vi "Big_LED_control.vi"() -> ()   [LabVIEW 2018]
uses:
  C:/Users/user/Desktop/LabVIEW/LED_CONTROL_big/LED_CONTROL_big_LED_ophir/AT lib/AmateurStepperMotor.dll
  AT lib/AmateurStepperMotor.dll
  <instrlib>/niDMM/nidmm.llb/niDMM Function.ctl
  <instrlib>/niDMM/nidmm.llb/niDMM Resolution in Digits.ctl
  <instrlib>/niDCPower/nidcpower.llb/niDCPower Measurement Type.ctl
  <vilib>/Instr/_visa.llb/VISA Configure Serial Port (Instr).vi
  <instrlib>/niDMM/nidmm.llb/niDMM Configure Measurement Digits.vi
panel:
  in  "Tab Control":T1(tab)
  in  "POWER":bool
  in  "Стоп":bool
  in  "Resource Name":refnum<k15>="PXI1Slot2" caption="Источник питания"
  in  "Амперметр":refnum<k15>="PXI1Slot5" caption="NI DMM 1"
  in  "V_MB, V":dbl=5.0 caption="voltage level" format="%_6p"
  in  "curlim_V_MB, A":dbl=0.3 caption="current limit" format="%_6p"
  in  "curlim_V_RESERVE, A":dbl=0.1 caption="current limit" min=0.01 format="%_6p"
  out "currentmes_V_MB, A":dbl caption="measurement" format="%_6g"
  out "currentmes_V_RESERVE, A":dbl caption="measurement" format="%_6g"
  in  "V_RESERVE, V":dbl caption="voltage level" format="%_6p"
  out "chart_2":dbl(graph)=8.556104343922883e-07
  out "chart_0":dbl(graph)=5.42616690347781e-05 caption="Waveform Chart 5"
  in  "curlim_V_LED, A":dbl=0.01 caption="current limit" min=0.01 format="%_6p"
  in  "V_LED, V":dbl=2.000000000000001 caption="voltage level" format="%_6p"
  out "chart_1":dbl(graph)=2.456762028615791e-06 caption="Waveform Chart 5"
  out "currentmes_V_LED, A":dbl caption="measurement" format="%_6g"
  in  "NI DMM 1 Current Range 3":string(combo)="1" caption="Range"
  in  "NI DMM 1 units 3":string(combo)="1000" caption="Units"
  out "Current Char":dbl(graph)=0.013612861948786303
  out "Current":dbl format="%_6g"
  in  "Arduino":refnum<visa-resource-name>="COM14"
  in  "Сегменты":bool[](array[boolean])=[FALSE, FALSE, FALSE, FALSE, FALSE, FALSE, FALSE, FALSE, FALSE, FALSE]
  in  "Вольтметр":refnum<k15>="PXI1Slot5" caption="NI DMM 1"
  in  "NI DMM 1 Voltage Range 4":string(combo)="-1" caption="Range"
  out "Voltage Char":dbl(graph)=0.013612861948786303
  in  "NI DMM 1 units 4":string(combo)="1" caption="Units"
  out "Voltage":dbl format="%_6g"
  out "Тип индикатора":string
  in  "Промер":bool caption="Промер сегмента"
  in  "Ophir 1 Info":u16(ring)=1 caption="Info" items=["Device : JUNO; s/n:903793", "Head : PD300R-3W   ; s/n:779628"]
  out "Ophir 1 Initialization":bool caption="Initialization"
  out "Position":dbl
  out "Готово":bool
  in  "Стоп GoTo":bool
  in  "Погнали!":bool
  in  "Speed":dbl=1000.0
  in  "StepDivisor":i32(ring)=8 items=["D1"=1, "D2"=2, "D4"=4, "D8"=8, "D16"=16, "D32"=32]
  in  "StepMultiplicationFactor":dbl=1.0
  in  "Ophir 1 Wait":u32=100 caption="Wait"
  in  "Ophir 1 Clear":bool caption="Clear"
  out "Ophir 1 MAX":dbl caption="MAX" format="%#_5g"
  out "Ophir 1 Optical Power":dbl caption="Power" format="%#_4g"
  out "Ophir 1 Over Range":bool caption="Over Range"
  in  "Ophir 1 units":string(combo)="1000" caption="Units"
  in  "HoldOn":bool
  in  "AccelerationTime, s":dbl
  in  "DecelerationTime, s":dbl
  out "Ophir 1 Char":dbl(graph)=6.67426339573744e-05
  in  "Go To":dbl
  in  "wave_lenght":string
  in  "Port Name":string="COM1"
  in  "measure path":path=path "D:/NI LabVIEW/MultiOpto/MultiOpto_1.2/Logs/SEL"
  in  "Сегмент":string caption="Введи сегмент"
  in  "Температура":string caption="Введи температуру"
  out "Образец №":string="0"
  out "Разряд":dbl
  out "+/-":bool
  out "Power off":bool
  in  "Ophir 1 error in (no error)":errorcluster caption="error in (no error)"
  out "Ophir 1 error out":errorcluster caption="error out"
  in  "Ophir 1 Select Communication Protocol":u16(ring) caption="Select Communication Protocol" items=["USB", "RS232", "GPIB"]
  in  "Ophir 1 Port Number (default 2)":i16=1 caption="Port Number (default 2)" min=0 max=20
  in  "Ophir 1 GPIB Address (10)":string="10" caption="GPIB Address (10)"
  out "Ophir 1 Real Optical Power":dbl format="%.6e"
  in  "Ophir 1 Baud Rate (3:9600)":i16(ring)=3 caption="Baud Rate (3:9600)" items=["300", "1200", "4800", "9600", "19200", "38400"]
  out "Ophir 1 dup Visa Session":refnum<visa-resource-name>="USB0::0x0BD3::0x0777::NI-VISA-10003::RAW" caption="dup Visa Session"
  in  "Ophir 1 usb channel":i16 caption="usb channel"
  in  "Command":string="led_on"
  in  "Записать":bool
  out "measure output file refnum":refnum<file>
  out "Device Response":string="*\n"
  out "Voltage, V":dbl caption="Measurement" format="%.5f"
  out "Current, A":dbl caption="Measurement" format="%.5f"
  # "V_MB 5 В\nогрничение 300 м\n\nV_LED 2,1 В\nограничение 200 м"
  # "единицы мА\nrange 1 А"
  # "единицы В\nrange AUTO"
  # "24.063\n\n     I          U\n20 мА  1.3 В\n20 мА  1.4 В\n 7 мА   1.15 В"
  # "24.064\n\n     I          U\n10 мА  2 В\n10 мА  2.15 В\n 7 мА   1.9 В"
  # "Р1:  +25°C\nР2:  - 60°C\nР3:  +85°C"
  # "j"
  # "c"
  # "d"
  # "e"
  # "g"
  # "h"
  # "a"
  # "b"
  # "f"
  # "k"
  # "L"
  # "m"
  # "n"
  # "p"
  # "dp"
  # "all"
  # "необходимо выдерживать 1 с между нажатиями кнопок"
  # "Шаговик"
  # "Офир"
  # "0. ввести номер образца\n1. включить нужный сегмент\n2. ввести его в поле справа\n3. вести температуру в поле слева\n4. нажать кнопку \"промер сегмента\""
  # "Введи ->"
  # "\"опрашивать кнопки не чаще, чем раз в секунду. сейчас кликать можно чаще, они загорятся, но ничего не произойдет\""
  # "Офир"
  # "автоматизировать подбор напряжения по известному максимальному напряжению и току. ОС по току сегмента"
  # "регклировка суммарного тока через индикатор"
  # "регулировать ток в зависимости от температуры.\nс ростом температуры растет ток.\nпид-регулятор??"
  # "1. каждый сегмент включаем по отдельности, резистором постраиваем ток до 10 мА\n2. напряжение V_LED при этом не меняется\n3. в такоом положении промеряем сегменты по отдельности\n4. для промера всего индикатора сразу подстраиваем напряжение при неизменном положении резисторов\n5. ток всех индикаторов = ток одного сегмента (10 мА) * число сегментов (15)\n6. добиваемся этого увеличением V_LED"
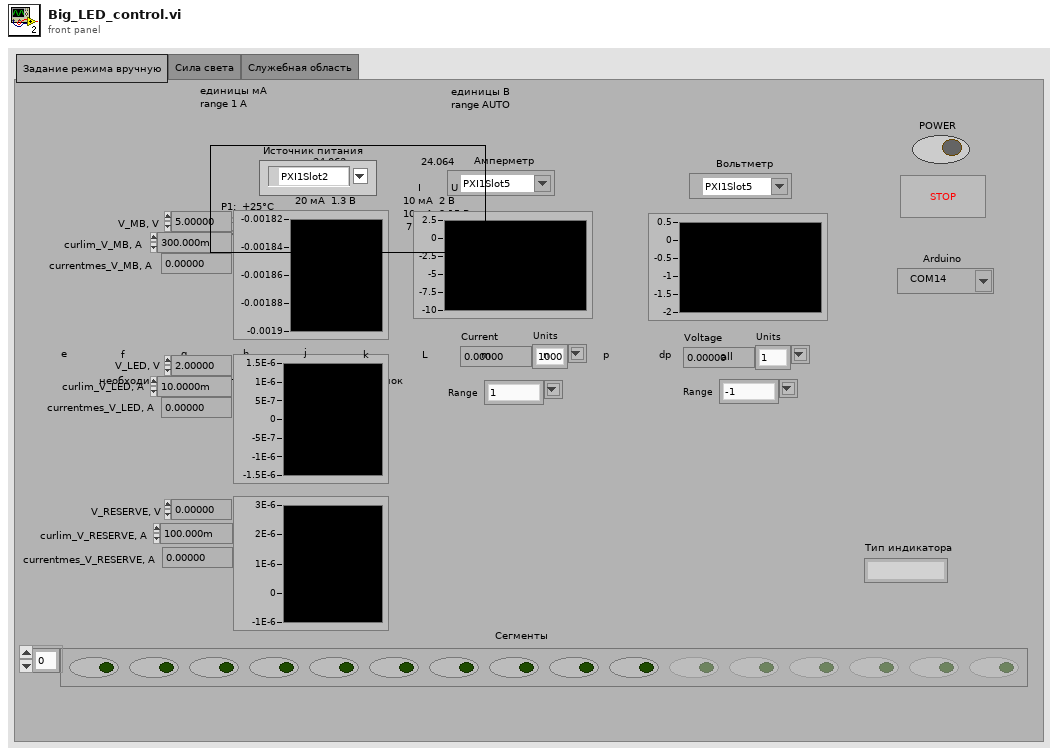
[diagram p1: front panel]
types:
  T1 = enum32{"Задание режима вручную", "Сила света", "Служебная область"}
  T2 = enum16{"open", "replace", "create", "open or create", "replace or create", "replace or create with confirmation"}
  T3 = typedef "niDCPower Measurement Type.ctl" = i32
  T4 = typedef "niDMM Function.ctl" = enum16{"DC Volts", "AC Volts", "DC Current", "AC Current", "2-wire Resistance", "4-wire Resistance", "Diode", "Frequency", "Period", "AC Volts DC Coupled", "Capacitance", "Inductance", "Temperature"}
  T5 = typedef "niDMM Resolution in Digits.ctl" = dbl
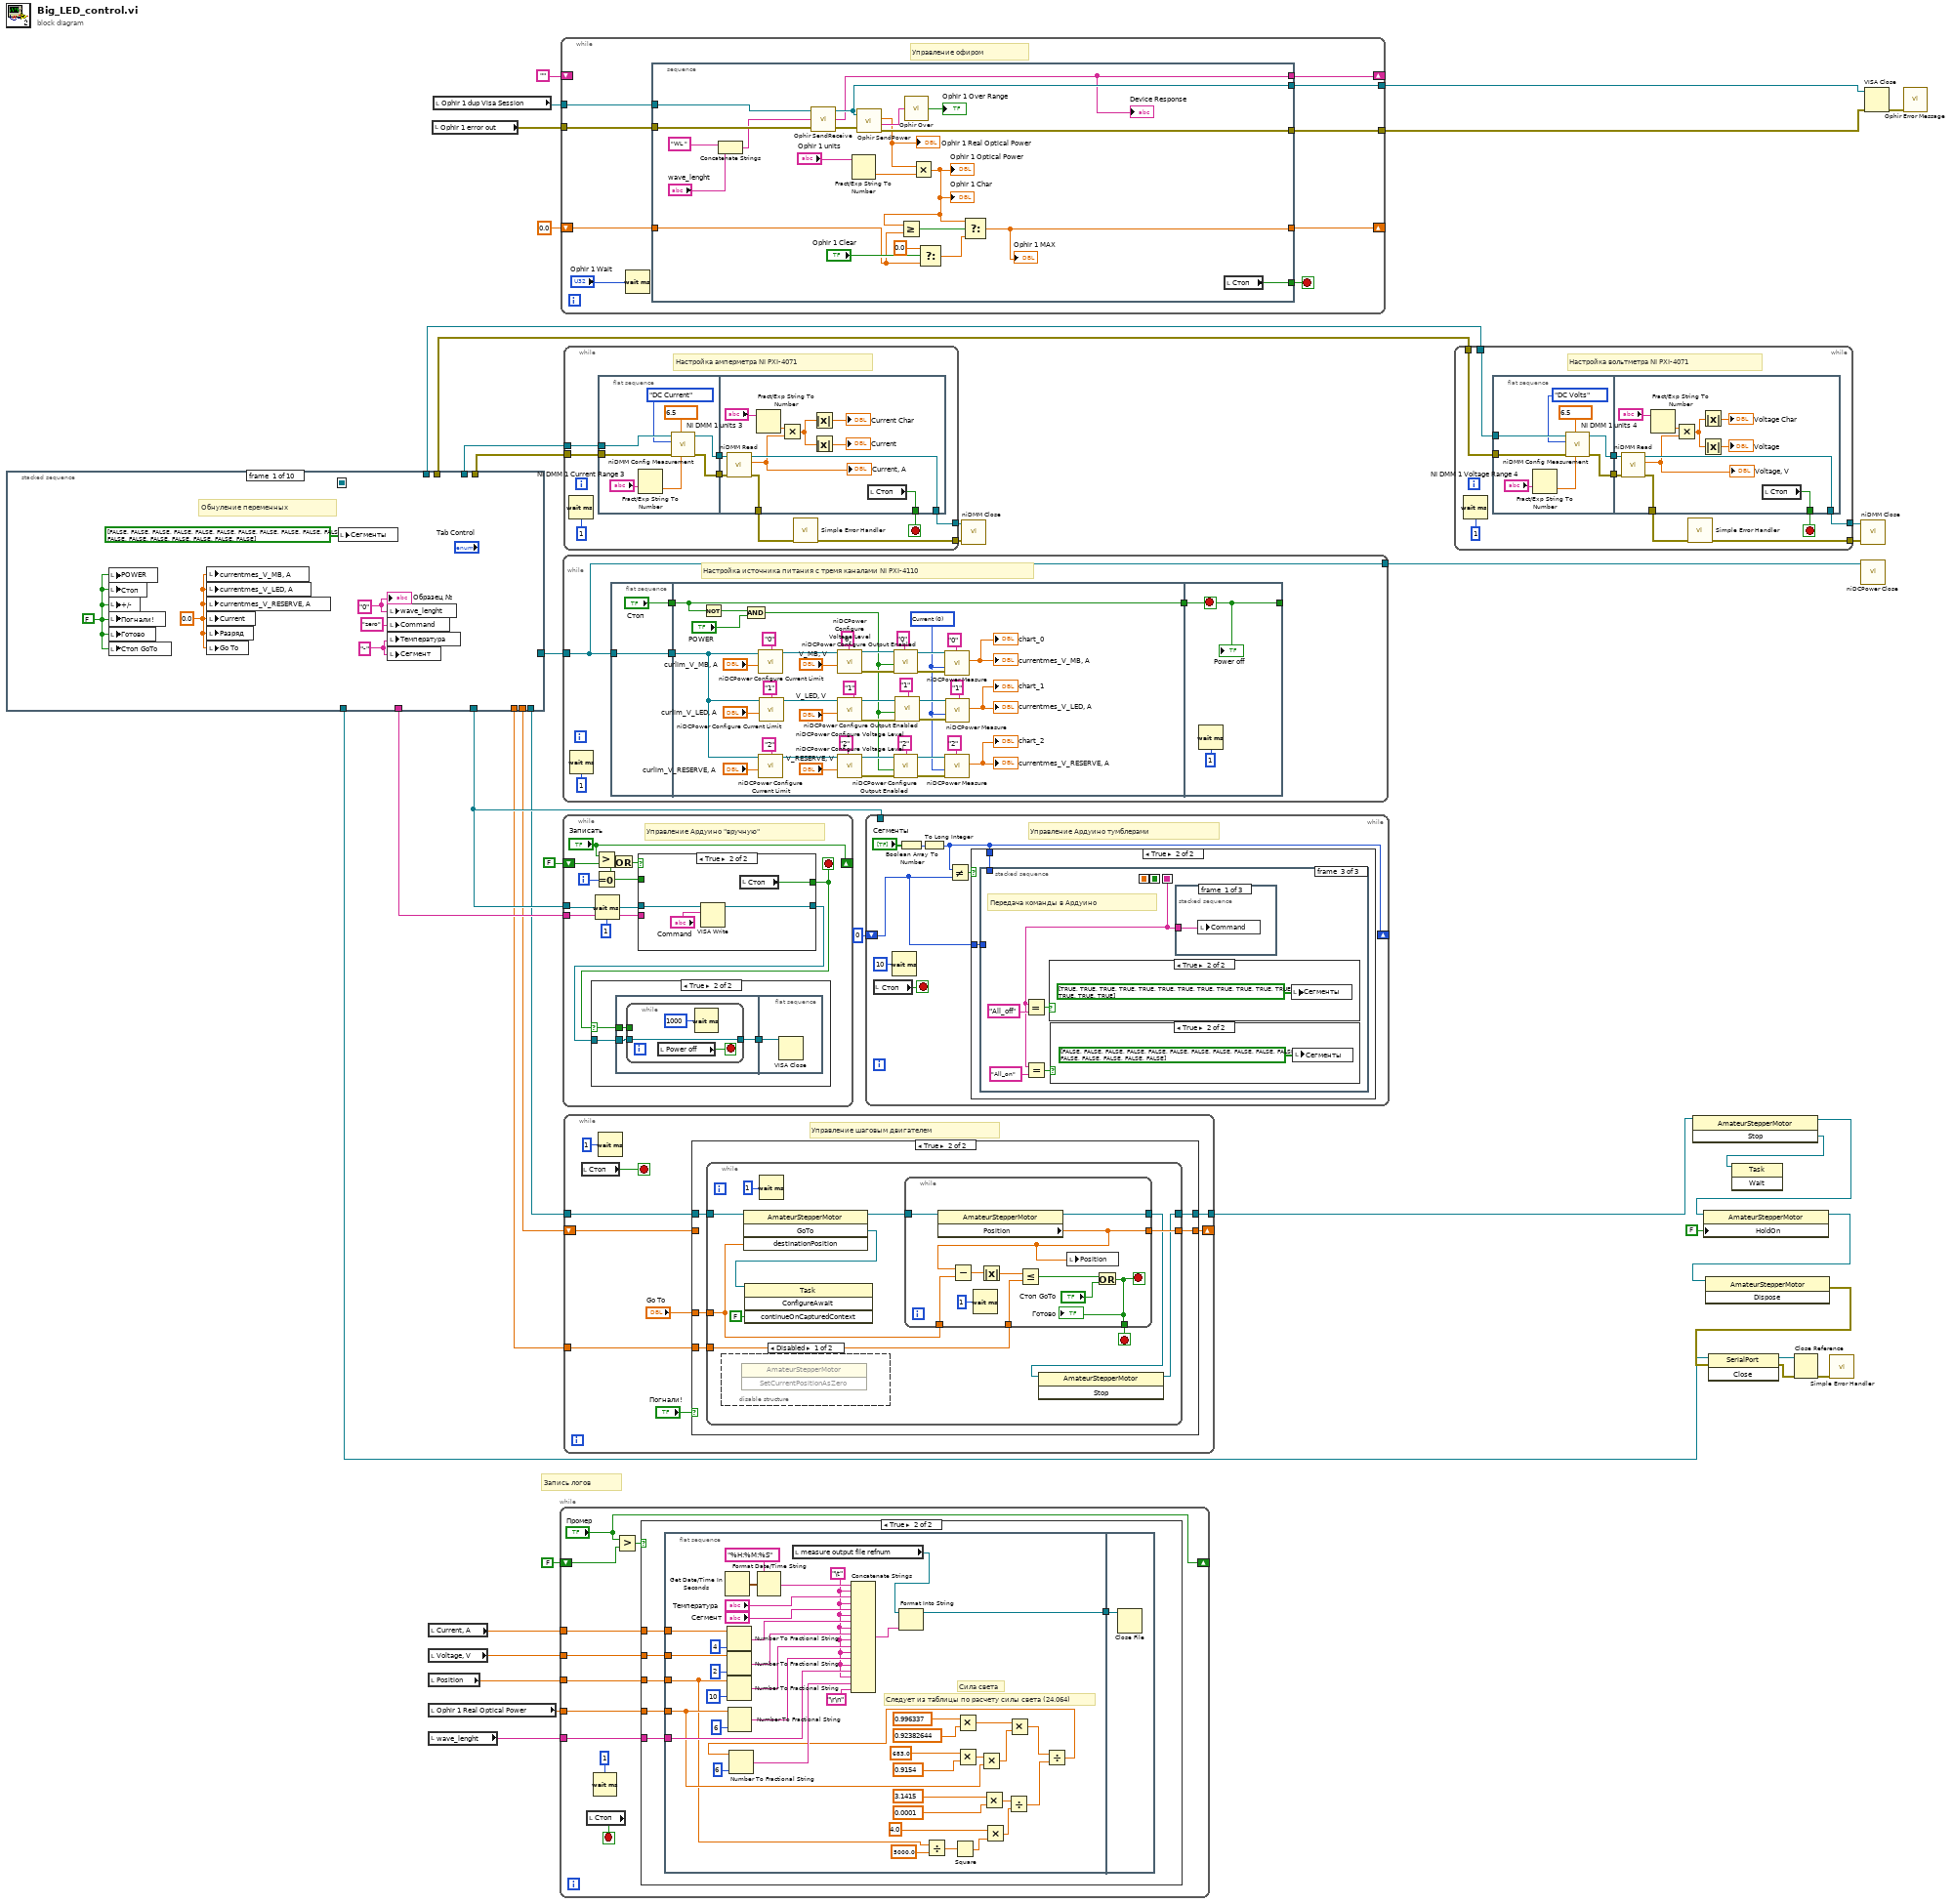
[diagram p0: block diagram]
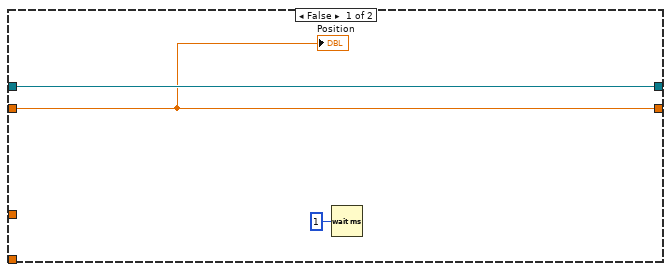
[diagram p3: hidden frame]
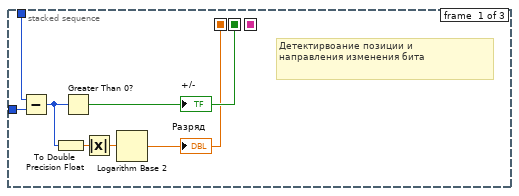
[diagram p6: hidden frame]
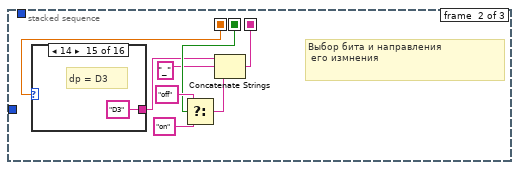
[diagram p7: hidden frame]
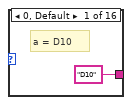
[diagram p8: hidden frame]
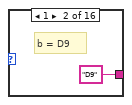
[diagram p9: hidden frame]
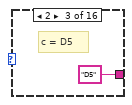
[diagram p10: hidden frame]
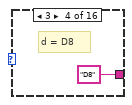
[diagram p11: hidden frame]
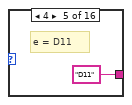
[diagram p12: hidden frame]
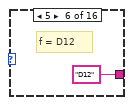
[diagram p13: hidden frame]
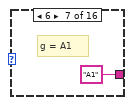
[diagram p14: hidden frame]
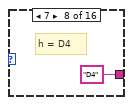
[diagram p15: hidden frame]
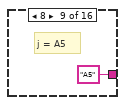
[diagram p16: hidden frame]
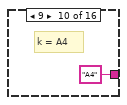
[diagram p17: hidden frame]
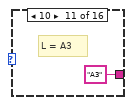
[diagram p18: hidden frame]
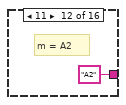
[diagram p19: hidden frame]
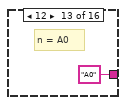
[diagram p20: hidden frame]
diagram:
  # "Запиcь логов"
  n1 = stacked-sequence {
    seq-local: [_ _ _ _ _ _ w82 _ _ _] -> [_ _ _ _ _ _ _ w94 _ _]
    tunnel: [_ _ _ w53 _ _ _ _ _ _] -> w28
    tunnel: [_ w49 _ _ _ _ _ _ _ _] -> w40
    tunnel: [_ w48 _ _ _ _ _ _ _ _] -> w39
    tunnel: [_ _ _ _ w59 _ _ _ _ _] -> w36
    tunnel: [_ _ _ _ _ _ _ _ _ w136] -> w35
    tunnel: [_ _ w52 _ _ _ _ _ _ _] -> w34
    tunnel: [_ _ w51 _ _ _ _ _ _ _] -> w33
    tunnel: [_ _ _ _ _ _ _ w97 _ _] -> w27
    tunnel: [_ _ _ _ _ _ _ w95 _ _] -> w25
    tunnel: [_ _ _ _ _ _ _ w96 _ _] -> w26
    tunnel: [_ _ _ _ _ _ w83 _ _ _] -> w9
    frame #0 {
      w42 = "-" ("Температура")
      w41 = "0" ("Образец №")
      w43 = 0.0 ("currentmes_2")
      w44 = FALSE ("Стоп")
      # "Обнуление переменных"
      n2 = local write "POWER"(w44) -> ()
      n3 = local write "Стоп"(w44) -> ()
      n4 = local write "+/-"(w44) -> ()
      n5 = local write "Погнали!"(w44) -> ()
      n6 = local write "Готово"(w44) -> ()
      n7 = local write "Стоп GoTo"(w44) -> ()
      n8 = local write "currentmes_V_MB, A"(w43) -> ()
      n9 = local write "currentmes_V_LED, A"(w43) -> ()
      n10 = local write "currentmes_V_RESERVE, A"(w43) -> ()
      n11 = local write "Current"(w43) -> ()
      n12 = local write "Разряд"(w43) -> ()
      n13 = local write "Go To"(w43) -> ()
      n14 = local write "Сегменты"(bool[] [FALSE, FALSE, FALSE, FALSE, FALSE, FALSE, FALSE, FALSE, FALSE, FALSE, FALSE, FALSE, FALSE, FALSE, FALSE, FALSE, FALSE, FALSE] ("Сегменты")) -> ()
      n15 = local write "wave_lenght"(w41) -> ()
      n16 = local write "Command"("zero" ("Command 2")) -> ()
      n17 = local write "Температура"(w42) -> ()
      n18 = local write "Сегмент"(w42) -> ()
      "Образец №" <- w41
    }
    frame #1 {
      # "Инициализация амперметра"
      n19 = call <instrlib>:"niDMM Initialize.vi"("Instrument Descriptor"="Амперметр") -> ("error out"=w49:errorcluster, "instrument handle out"=w48:refnum<k15>)  [unwired: 9 in]
    }
    frame #2 {
      # "Инициализация вольтметра"
      n20 = call <instrlib>:"niDMM Initialize.vi"("Instrument Descriptor"="Вольтметр") -> ("error out"=w51:errorcluster, "instrument handle out"=w52:refnum<k15>)  [unwired: 9 in]
    }
    frame #3 {
      # "Инициализация источника питания"
      n21 = call <instrlib>:"niDCPower Initialize.vi"("resource name"="Resource Name") -> ("error out"=w55:errorcluster, "instrument handle out"=w56:refnum<k15>)  [unwired: 3 in, 6 out]
      n22 = call <instrlib>:"niDCPower Configure Voltage Level.vi"("error in (no error)"=w55, "voltage level"=0.0, "channel name"="0,1,2", "instrument handle"=w56) -> ("instrument handle out"=w53:refnum<k15>)  [unwired: 6 in, 1 out]
    }
    frame #4 {
      # "Инициализация Ардуино"
      n23 = call-poly "VISA Configure Serial Port"("VISA resource name"="Arduino", "baud rate (9600)"=u32 9600) -> ("VISA resource name out"=w59:refnum<visa-resource-name>)  [unwired: 12 in, 1 out]
    }
    frame #5 {
      # "Инициализация офира"
      n24 = call "Ophir InitCom.vi"("GPIB Address (default 10)"="Ophir 1 GPIB Address (10)", "Communication (default USB 0)"="Ophir 1 Select Communication Protocol", "USB Channel number (default 0)"="Ophir 1 usb channel", "Port Number (default 2)"="Ophir 1 Port Number (default 2)", "error in (no error)"="Ophir 1 error in (no error)", "Baud Rate (3:9600)"="Ophir 1 Baud Rate (3:9600)") -> ("dup Visa Session"=w68:refnum<visa-resource-name>, "error out"=w67:errorcluster)  [unwired: 1 out]
      n25 = call "Ophir InstrInfo.vi"("Visa Session"=w68, "error in (no error)"=w67) -> ("dup Visa Session"=w80:refnum<visa-resource-name>, "Instrument Info"=w62:string, "error out"=w78:errorcluster)
      n26 = call "Ophir HeadInfo.vi"("Visa Session"=w80, "error in (no error)"=w78) -> ("error out"=w77:errorcluster, "dup Visa Session"=w79:refnum<visa-resource-name>, "Head Info"=w76:string)  [unwired: 6 out]
      n27 = call "Ophir InfoStrings.vi"("error in (no error)"=w77, "Head Info"=w76, "Instrument Info"=w62) -> ("error out"=w75:errorcluster, "Strings Array"=w74:string[])
      n28 = property on="Ophir 1 Info" class="Ring (strict)"("Strings []"=w74) -> ()  [unwired: 2 in, 2 out]
      n29 = call "Ophir ConfigDevice.vi"("Visa Session"=w79, "Measure Choice (0:Power)"=u16 0, "error in (no error)"=w75) -> ("dup Visa Session"=→"Ophir 1 dup Visa Session":refnum<visa-resource-name>, "OK ?"=→"Ophir 1 Initialization":bool, "error out"=→"Ophir 1 error out":errorcluster)  [unwired: 1 out]
    }
    frame #6 {
      w86 = 100 ("WriteTimeout")
      w93 = 1 items=["None", "One", "Two", "OnePointFive"] ("stopBits")
      w90 = 0 items=["None", "Odd", "Even", "Mark", "Space"] ("parity")
      # "Инициализация шаговика ч.1"
      n30 = constructor class="SerialPort"("portName"="Port Name", "baudRate"=57600, "parity"=w90, "dataBits"=8, "stopBits"=w93) -> (reference out=w88:refnum<k24>, error out=w87:errorcluster)  [unwired: 3 in, 6 out]
      n31 = invoke class="SerialPort" method="Open"(reference=w88, error in=w87) -> (reference out=w85:refnum<k24>, error out=w84:errorcluster)  [unwired: 1 in, 1 out]
      n32 = property class="SerialPort"(reference=w85, "WriteTimeout"=w86, "ReadTimeout"=w86) -> (reference out=w83:refnum<k24>)  [unwired: 1 in, 1 out]
      n33 = constructor class="AmateurStepperMotor"(error in=w84, "serialPort"=w83) -> (reference out=w82:refnum<k24>)  [unwired: 2 in, 3 out]
    }
    frame #7 {
      # "Инициализация шаговика ч.2"
      n34 = property class="AmateurStepperMotor"(reference=w94, "Speed"="Speed", "StepDivisor"="StepDivisor", "StepMultiplicationFactor"="StepMultiplicationFactor", "AccelerationTime"="AccelerationTime, s", "DecelerationTime"="DecelerationTime, s", "HoldOn"="HoldOn") -> (reference out=w97:refnum<k24>, "Position"=w95:dbl, "PositioningPrecision"=w96:dbl)  [unwired: 1 in, 1 out]
    }
    frame #8 {
      w106 = "\t"
      # "Инициализация логов"
      n35 = local read "Образец №"() -> (w130:string)
      n36 = Get Date/Time In Seconds() -> (seconds since 1Jan1904=w124:timestamp)
      n37 = Build Path(base path="measure path", name or relative path=w130) -> (appended path=w120:path)
      n38 = call <vilib>:"Check if File or Folder Exists.vi"("path"=w120) -> ("file or folder exists?"=w121:bool, "dup path"=w122:path)  [unwired: 8 in, 1 out]
      n39 = Format Date/Time String(time format string (%c)="MES %d %m %y %H.%M.%S", seconds (now)=w124) -> (date/time string=w125:string)  [unwired: 1 in]
      n40 = case shown="False" w121 {
        tunnel: w122 -> [w134 w135]
        tunnel: [w133 w135] -> w123
        frame False {
          n41 = Create Folder(path (use dialog)=w134) -> (created path=w133:path)  [unwired: 2 in, 2 out]
        }
        frame True {
        }
      }
      n42 = Concatenate Strings(w125, ".xls" ("string")) -> (w126:string)
      n43 = Build Path(base path=w123, name or relative path=w126) -> (appended path=w127:path)
      n44 = Open/Create/Replace File(file path (use dialog)=w127, operation (0:open)=T2."open or create", access (0:read/write)=enum16{"read/write", "read-only", "write-only"}."read/write") -> (refnum out=w128:refnum<file>)  [unwired: 3 in, 2 out]
      n45 = Set File Position(refnum=w128, from (0:start)=enum16{"start", "end", "current"}."end") -> (refnum out=w131:refnum<file>)  [unwired: 2 in, 1 out]
      n46 = Format Into String(initial string=w131, "Time" ("string"), w106, "Temperature, C" ("string"), w106, "Segment" ("string"), w106, "Current, mA" ("string"), w106, "Voltage, V" ("input 7"), w106, "Distance, m" ("string"), w106, "Power, W " ("string"), w106, "Wavelenght, nm" ("input 17"), w106, "Candlepower, kd" ("string"), "\r\n") -> (resulting string=→"measure output file refnum":refnum<file>)  [unwired: 2 in, 1 out]
    }
    frame #9 {
      # "Begin VI: ОК или ОА?"
      n47 = call "Begin.vi"() -> ("String"=w136:string)  [unwired: 8 in]
      "Тип индикатора" <- w136
      n48 = local write "Command"(w136) -> ()
    }
  }
  n49 = local read "Current, A"() -> (w6:dbl)
  n50 = local read "Voltage, V"() -> (w5:dbl)
  n51 = local read "Position"() -> (w4:dbl)
  n52 = local read "Ophir 1 Real Optical Power"() -> (w3:dbl)
  n53 = local read "wave_lenght"() -> (w2:string)
  n54 = local read "Ophir 1 error out"() -> (w23:errorcluster)
  n55 = local read "Ophir 1 dup Visa Session"() -> (w24:refnum<visa-resource-name>)
  n56 = while {
    tunnel: w6 -> [w146]
    tunnel: w5 -> [w145]
    tunnel: w4 -> [w144]
    tunnel: w3 -> [w143]
    tunnel: w2 -> [w142]
    shift-right: ["Промер"] -> _
    shift-left: FALSE ("Промер сегмента") -> [w139]
    stop <- w137 stop-if-true
    n57 = local read "Стоп"() -> (w137:bool)
    n58 = Wait (ms)(milliseconds to wait=u32 1) -> ()  [unwired: 1 out]
    n59 = Greater?(x="Промер", y=w139) -> (0:w140:bool)
    n60 = case shown="True" w140 {
      tunnel: w146 -> [_ w152]
      tunnel: w145 -> [_ w151]
      tunnel: w144 -> [_ w148]
      tunnel: w143 -> [_ w149]
      tunnel: w142 -> [_ w150]
      frame False {
      }
      frame True {
        n61 = flat-sequence {
          tunnel: w152 -> [w185]
          tunnel: w151 -> [w184]
          tunnel: w150 -> [w182]
          tunnel: w149 -> [w171]
          tunnel: w148 -> [w161]
          tunnel: [w153] -> w147
          tunnel: w147 -> [w196]
          frame #0 {
            w181 = "\t"
            # "Сила света"
            # "Следует из таблицы по расчету силы света (24.064)"
            n62 = Get Date/Time In Seconds() -> (seconds since 1Jan1904=w195:timestamp)
            n63 = Number To Fractional String(number=w185, precision (6)=i16 4) -> (F-format string=w188:string)  [unwired: 2 in]
            n64 = Number To Fractional String(number=w184, precision (6)=i16 2) -> (F-format string=w187:string)  [unwired: 2 in]
            n65 = Number To Fractional String(number=w161, precision (6)=i16 10) -> (F-format string=w186:string)  [unwired: 2 in]
            n66 = Number To Fractional String(number=w171, precision (6)=i16 6) -> (F-format string=w183:string)  [unwired: 2 in]
            n67 = Format Date/Time String(time format string (%c)="%H:%M:%S", seconds (now)=w195) -> (date/time string=w193:string)  [unwired: 1 in]
            n68 = local read "measure output file refnum"() -> (w189:refnum<file>)
            n69 = Divide(x=w161, y=5000.0) -> (x/y=w163:dbl)
            n70 = Square(x=w163) -> (x^2=w162:dbl)
            n71 = Multiply(x=0.996337, y=0.92382644) -> (x*y=w177:dbl)
            n72 = Multiply(x=683.0, y=0.9154) -> (x*y=w172:dbl)
            n73 = Multiply(x=w172, y=w171) -> (x*y=w170:dbl)
            n74 = Multiply(x=3.1415, y=0.0001) -> (x*y=w166:dbl)
            n75 = Multiply(x=4.0, y=w162) -> (x*y=w165:dbl)
            n76 = Divide(x=w166, y=w165) -> (x/y=w167:dbl)
            n77 = Multiply(x=w177, y=w170) -> (x*y=w176:dbl)
            n78 = Divide(x=w176, y=w167) -> (x/y=w159:dbl)
            n79 = Number To Fractional String(number=w159, precision (6)=i16 6) -> (F-format string=w175:string)  [unwired: 2 in]
            n80 = Concatenate Strings(w193, w181, "Температура", w181, "Сегмент", w181, w188, w181, w187, w181, w186, w181, w183, w181, w182, w181, w175, "\r\n") -> (w190:string)
            n81 = Format Into String(initial string=w189, w190) -> (resulting string=w153:refnum<file>)  [unwired: 2 in, 1 out]
          }
          frame #1 {
            n82 = Close File(refnum=w196) -> ()  [unwired: 1 in, 2 out]
          }
        }
      }
    }
  }
  n83 = while {
    tunnel: [w205] -> w19
    tunnel: [w199] -> w20
    tunnel: w24 -> [w203]
    tunnel: w23 -> [w202]
    shift-right: [w200] -> _
    shift-left: 0.0 ("t") -> [w201]
    shift-right: [w197] -> _
    shift-left: "" -> [_]
    stop <- w204 stop-if-true
    # "Управление офиром"
    n84 = Wait (ms)(milliseconds to wait="Ophir 1 Wait") -> ()  [unwired: 1 out]
    n85 = stacked-sequence {
      tunnel: [w227] -> w205
      tunnel: [w214] -> w204
      tunnel: w203 -> [w211]
      tunnel: w202 -> [w210]
      tunnel: w201 -> [w218]
      tunnel: [w216] -> w200
      tunnel: [w212] -> w199
      tunnel: [w206] -> w197
      frame #0 {
        n86 = Concatenate Strings("WL " ("string"), "wave_lenght") -> (w207:string)
        n87 = call "Ophir SendReceive.vi"("error in (no error)"=w210, "Command"=w207, "Visa Session"=w211) -> ("error out"=w213:errorcluster, "Frame Output"=w206:string, "dup Visa Session"=w212:refnum<visa-resource-name>)
        "Device Response" <- w206
        n88 = Fract/Exp String To Number(string="Ophir 1 units") -> (number=w217:dbl)  [unwired: 3 in, 1 out]
        n89 = call "Ophir SendPower.vi"("Visa Session"=w212, "error in (no error)"=w213) -> ("Value Number"=w215:dbl, "Value String"=w225:string, "error out"=w227:errorcluster)  [unwired: 1 out]
        "Ophir 1 Real Optical Power" <- w215
        n90 = call "Ophir Over.vi"("Value String"=w225) -> ("Overrange"=→"Ophir 1 Over Range":bool)
        n91 = Multiply(x=w215, y=w217) -> (x*y=w222:dbl)
        "Ophir 1 Char" <- w222
        "Ophir 1 Optical Power" <- w222
        n92 = Greater Or Equal?(x=w222, y=w218) -> (x >= y?=w223:bool)
        n93 = Select(t=0.0, s="Ophir 1 Clear", f=w218) -> (s? t:f=w221:dbl)
        n94 = Select(t=w222, s=w223, f=w221) -> (s? t:f=w216:dbl)
        "Ophir 1 MAX" <- w216
        n95 = local read "Стоп"() -> (w214:bool)
      }
    }
  }
  n96 = while {
    tunnel: w28 -> [w229]
    tunnel: [w229] -> w37
    stop <- w230 stop-if-true
    # "Настройка источника питания с тремя каналами NI PXI-4110"
    n97 = Wait (ms)(milliseconds to wait=u32 1) -> ()  [unwired: 1 out]
    n98 = flat-sequence {
      tunnel: w229 -> [w235]
      tunnel: [w235] -> w232
      tunnel: ["Стоп"] -> w231
      tunnel: w232 -> [w243]
      tunnel: w231 -> [w277]
      tunnel: [w277] -> w228
      tunnel: [w279] -> w230
      tunnel: w228 -> [w279]
      frame #0 {
      }
      frame #1 {
        w242 = T3 0 items=["Current", "Voltage"] ("measurement type")
        n99 = Not(x=w277) -> (.not. x?=w276:bool)
        n100 = And(x=w276, y="POWER") -> (x .and. y?=w238:bool)
        n101 = call <instrlib>:"niDCPower Configure Current Limit.vi"("current limit"="curlim_V_MB, A", "channel name"="0", "instrument handle"=w243) -> ("instrument handle out"=w262:refnum<k15>)  [unwired: 7 in, 1 out]
        n102 = call <instrlib>:"niDCPower Configure Current Limit.vi"("current limit"="curlim_V_RESERVE, A", "channel name"="2", "instrument handle"=w243) -> ("instrument handle out"=w261:refnum<k15>)  [unwired: 7 in, 1 out]
        n103 = call <instrlib>:"niDCPower Configure Current Limit.vi"("current limit"="curlim_V_LED, A", "channel name"="1", "instrument handle"=w243) -> ("instrument handle out"=w270:refnum<k15>)  [unwired: 7 in, 1 out]
        n104 = call <instrlib>:"niDCPower Configure Voltage Level.vi"("voltage level"="V_MB, V", "channel name"="0", "instrument handle"=w262) -> ("error out"=w267:errorcluster, "instrument handle out"=w264:refnum<k15>)  [unwired: 7 in]
        n105 = call <instrlib>:"niDCPower Configure Voltage Level.vi"("voltage level"="V_LED, V", "channel name"="1", "instrument handle"=w270) -> ("error out"=w273:errorcluster, "instrument handle out"=w271:refnum<k15>)  [unwired: 7 in]
        n106 = call <instrlib>:"niDCPower Configure Voltage Level.vi"("voltage level"="V_RESERVE, V", "channel name"="2", "instrument handle"=w261) -> ("error out"=w266:errorcluster, "instrument handle out"=w265:refnum<k15>)  [unwired: 7 in]
        n107 = call <instrlib>:"niDCPower Configure Output Enabled.vi"("error in (no error)"=w267, "output enabled"=w238, "channel name"="0", "instrument handle"=w264) -> ("error out"=w257:errorcluster, "instrument handle out"=w258:refnum<k15>)  [unwired: 6 in]
        n108 = call <instrlib>:"niDCPower Configure Output Enabled.vi"("error in (no error)"=w266, "output enabled"=w238, "channel name"="2", "instrument handle"=w265) -> ("error out"=w256:errorcluster, "instrument handle out"=w255:refnum<k15>)  [unwired: 6 in]
        n109 = call <instrlib>:"niDCPower Configure Output Enabled.vi"("error in (no error)"=w273, "output enabled"=w238, "channel name"="1", "instrument handle"=w271) -> ("error out"=w274:errorcluster, "instrument handle out"=w272:refnum<k15>)  [unwired: 6 in]
        n110 = call <instrlib>:"niDCPower Measure.vi"("error in (no error)"=w257, "measurement type"=w242, "channel name"="0", "instrument handle"=w258) -> ("measurement"=→"currentmes_V_MB, A" →"chart_0":dbl)  [unwired: 5 in, 2 out]
        n111 = call <instrlib>:"niDCPower Measure.vi"("error in (no error)"=w256, "measurement type"=w242, "channel name"="2", "instrument handle"=w255) -> ("measurement"=→"currentmes_V_RESERVE, A" →"chart_2":dbl)  [unwired: 5 in, 2 out]
        n112 = call <instrlib>:"niDCPower Measure.vi"("error in (no error)"=w274, "measurement type"=w242, "channel name"="1", "instrument handle"=w272) -> ("measurement"=→"chart_1" →"currentmes_V_LED, A":dbl)  [unwired: 5 in, 2 out]
      }
      frame #2 {
        n113 = Wait (ms)(milliseconds to wait=u32 1) -> ()  [unwired: 1 out]
        "Power off" <- w279
      }
    }
  }
  n114 = while {
    tunnel: w36 -> [w287]
    shift-right: ["Записать"] -> _
    shift-left: FALSE ("Записать") -> [w289]
    tunnel: w35 -> [w285]
    i -> [w286]
    stop <- w280 stop-if-true
    # "Управление Ардуино \"вручную\""
    n115 = Greater?(x="Записать", y=w289) -> (0:w283:bool)
    n116 = Equal To 0?(x=w286) -> (x = 0?=w282:bool)
    n117 = Wait (ms)(milliseconds to wait=u32 1) -> ()  [unwired: 1 out]
    n118 = Or(x=w283, y=w282) -> (x .or. y?=w284:bool)
    n119 = case shown="True" w284 {
      tunnel: w287 -> [w301 w306]
      tunnel: [w302 w305] -> w280
      tunnel: w285 -> [_ _]
      tunnel: w282 -> [_ _]
      tunnel: [w301 w303] -> w281
      frame False {
        n120 = local read "Стоп"() -> (w302:bool)
      }
      frame True {
        n121 = VISA Write(VISA resource name=w306, write buffer="Command") -> (VISA resource name out=w303:refnum<visa-resource-name>)  [unwired: 1 in, 2 out]
        n122 = local read "Стоп"() -> (w305:bool)
      }
    }
    n123 = case shown="True" w280 {
      selector: w280 -> [_ w291]
      tunnel: w281 -> [_ w293]
      frame False {
      }
      frame True {
        n124 = flat-sequence {
          tunnel: w293 -> [w296]
          tunnel: [w295] -> w292
          tunnel: w291 -> [w294]
          tunnel: w292 -> [w300]
          frame #0 {
            n125 = while {
              tunnel: w296 -> [w299]
              tunnel: [w299] -> w295
              tunnel: w294 -> [_]
              stop <- w297 stop-if-true
              n126 = local read "Power off"() -> (w297:bool)
              n127 = Wait (ms)(milliseconds to wait=u32 1000) -> ()  [unwired: 1 out]
            }
          }
          frame #1 {
            n128 = VISA Close(VISA resource name=w300) -> ()  [unwired: 1 in, 1 out]
          }
        }
      }
    }
  }
  n129 = while {
    tunnel: [w313] -> w29
    tunnel: w39 -> [w311]
    tunnel: w40 -> [w310]
    tunnel: [w307] -> w30
    stop <- w309 stop-if-true
    # "Настройка амперметра NI PXI-4071"
    n130 = Wait (ms)(milliseconds to wait=u32 1) -> ()  [unwired: 1 out]
    n131 = flat-sequence {
      tunnel: [w320] -> w315
      tunnel: w311 -> [w318]
      tunnel: w310 -> [w322]
      tunnel: [w319] -> w314
      tunnel: w315 -> [w331]
      tunnel: w314 -> [w334]
      tunnel: [w330] -> w309
      tunnel: [w329] -> w307
      tunnel: [w328] -> w308
      frame #0 {
        w316 = T5 6.5 items=["3 1/2"=3.5, "4 1/2"=4.5, "5 1/2"=5.5, "6 1/2"=6.5, "7 1/2"=7.5] ("Resolution in Digits")
        n132 = Fract/Exp String To Number(string="NI DMM 1 Current Range 3") -> (number=w321:dbl)  [unwired: 3 in, 1 out]
        n133 = call-poly <instrlib>:"niDMM Config Measurement.vi"("Range"=w321, "Resolution in Digits"=w316, "error in (no error)"=w322, "Function"=niDMM_Function."DC Current" ("Measurement Type"), "instrument handle"=w318) -> ("error out"=w319:errorcluster, "instrument handle out"=w320:refnum<k15>)  [unwired: 5 in]
      }
      frame #1 {
        n134 = call <instrlib>:"niDMM Read.vi"("error in (no error)"=w334, "instrument handle"=w331) -> ("error out"=w328:errorcluster, "Measurement"=w324:dbl, "instrument handle out"=w329:refnum<k15>)  [unwired: 7 in]
        "Current, A" <- w324
        n135 = Fract/Exp String To Number(string="NI DMM 1 units 3") -> (number=w332:dbl)  [unwired: 3 in, 1 out]
        n136 = Multiply(x=w332, y=w324) -> (x*y=w325:dbl)
        n137 = Absolute Value(x=w325) -> (abs(x)=→"Current Char":dbl)
        n138 = Absolute Value(x=w325) -> (abs(x)=→"Current":dbl)
        n139 = local read "Стоп"() -> (w330:bool)
      }
    }
    n140 = call <vilib>:"Simple Error Handler.vi"("error in (no error)"=w308) -> ("error out"=w313:errorcluster)  [unwired: 1 in, 7 out]
  }
  n141 = while {
    tunnel: w27 -> [w343]
    tunnel: w26 -> [w340]
    shift-right: [w339] -> _
    shift-left: w25 -> [w342]
    tunnel: [w338] -> w16
    stop <- w336 stop-if-true
    # "Управление шаговым двигателем"
    n142 = local read "Стоп"() -> (w336:bool)
    n143 = Wait (ms)(milliseconds to wait=u32 1) -> ()  [unwired: 1 out]
    n144 = case shown="True" "Погнали!" {
      tunnel: "Go To" -> [_ w351]
      tunnel: w343 -> [w345 w350]
      tunnel: [w345 w349] -> w338
      tunnel: w342 -> [w344 _]
      tunnel: [w344 w348] -> w339
      tunnel: w340 -> [_ w347]
      frame False {
        n145 = Wait (ms)(milliseconds to wait=u32 1) -> ()  [unwired: 1 out]
        "Position" <- w344
      }
      frame True {
        n146 = while {
          tunnel: w351 -> [w357]
          tunnel: w350 -> [w358]
          tunnel: [w354] -> w349
          tunnel: [w362] -> w348
          tunnel: w347 -> [w360]
          stop <- w361 stop-if-true
          n147 = disable-structure shown="Disabled" {
            frame Disabled {
              n148 = invoke class="AmateurStepperMotor" method="SetCurrentPositionAsZero"() -> ()  [unwired: 3 in, 3 out]
            }
            frame Enabled {
            }
          }
          n149 = invoke class="AmateurStepperMotor" method="GoTo"(reference=w358, "destinationPosition"=w357) -> (reference out=w352:refnum<k24>, "GoTo"=w356:refnum<k24>)  [unwired: 2 in, 2 out]
          n150 = invoke class="Task" method="ConfigureAwait"(reference=w356, "continueOnCapturedContext"=FALSE) -> ()  [unwired: 2 in, 4 out]
          n151 = Wait (ms)(milliseconds to wait=u32 1) -> ()  [unwired: 1 out]
          n152 = while {
            tunnel: [w365] -> w362
            tunnel: [w364] -> w353
            tunnel: [w367] -> w361
            tunnel: w357 -> [w372]
            tunnel: w360 -> [w370]
            tunnel: w352 -> [w363]
            stop <- w367 stop-if-true
            n153 = property class="AmateurStepperMotor"(reference=w363) -> (reference out=w364:refnum<k24>, "Position"=w365:dbl)  [unwired: 1 in, 1 out]
            n154 = Subtract(x=w365, y=w372) -> (x-y=w373:dbl)
            n155 = Wait (ms)(milliseconds to wait=u32 1) -> ()  [unwired: 1 out]
            n156 = Absolute Value(x=w373) -> (abs(x)=w371:dbl)
            n157 = Less Or Equal?(x=w371, y=w370) -> (x <= y?=w369:bool)
            n158 = local write "Position"(w365) -> ()
            n159 = Or(x=w369, y="Стоп GoTo") -> (x .or. y?=w367:bool)
            "Готово" <- w367
          }
          n160 = invoke class="AmateurStepperMotor" method="Stop"(reference=w353) -> (reference out=w354:refnum<k24>)  [unwired: 2 in, 2 out]
        }
      }
    }
  }
  n161 = while {
    shift-right: [w376] -> _
    shift-left: 0 -> [w377]
    tunnel: w36 -> [_]
    stop <- w380 stop-if-true
    # "Управление Ардуино тумблерами"
    n162 = local read "Стоп"() -> (w380:bool)
    n163 = Wait (ms)(milliseconds to wait=u32 10 ("millisecond timer value")) -> ()  [unwired: 1 out]
    n164 = Boolean Array To Number(Boolean array="Сегменты") -> (number=w375:u32)
    n165 = To Long Integer(number=w375) -> (32bit integer=w376:i32)
    n166 = Not Equal?(x=w376, y=w377) -> (x != y?=w378:bool)
    n167 = case shown="True" w378 {
      tunnel: w376 -> [_ w381]
      tunnel: w377 -> [_ w382]
      frame False {
      }
      frame True {
        n168 = stacked-sequence {
          seq-local: [w385 _ _] -> [_ w395 _]
          seq-local: [w383 _ _] -> [_ w390 _]
          seq-local: [_ w391 _] -> [_ _ w415]
          tunnel: w381 -> [w387 _ _]
          tunnel: w382 -> [w386 _ _]
          frame #0 {
            # "Детектирвоание позиции и\nнаправления изменения бита"
            n169 = Subtract(x=w387, y=w386) -> (x-y=w388:i32)
            n170 = To Double Precision Float(number=w388) -> (double precision float=w389:dbl)
            n171 = Greater Than 0?(x=w388) -> (x > 0?=w385:bool)
            "+/-" <- w385
            n172 = Absolute Value(x=w389) -> (abs(x)=w384:dbl)
            n173 = Logarithm Base 2(1:w384) -> (0:w383:dbl)
            "Разряд" <- w383
          }
          frame #1 {
            # "Выбор бита и направления\n его измнения"
            n174 = case shown="14" w390 {
              tunnel: ["D10" "D9" "D5" "D8" "D11" "D12" "A1" "D4" "A5" "A4" "A3" "A2" "A0" "D13" "D3" "All"] -> w393
              frame 0, Default {
                # "a = D10"
              }
              frame 1 {
                # "b = D9"
              }
              frame 2 {
                # "c = D5"
              }
              frame 3 {
                # "d = D8"
              }
              frame 4 {
                # "e = D11"
              }
              frame 5 {
                # "f = D12"
              }
              frame 6 {
                # "g = A1"
              }
              frame 7 {
                # "h = D4"
              }
              frame 8 {
                # "j = A5"
              }
              frame 9 {
                # "k = A4"
              }
              frame 10 {
                # "L = A3"
              }
              frame 11 {
                # "m = A2"
              }
              frame 12 {
                # "n = A0"
              }
              frame 13 {
                # "p = D13"
              }
              frame 14 {
                # "dp = D3"
              }
              frame 15 {
              }
            }
            n175 = Select(t="off", s=w395, f="on") -> (s? t:f=w392:string)
            n176 = Concatenate Strings(w393, "_" ("string"), w392) -> (w391:string)
          }
          frame #2 {
            # "Передача команды в Ардуино"
            n177 = Equal?(x=w415, y="All_off") -> (x = y?=w418:bool)
            n178 = Equal?(x=w415, y="All_on") -> (x = y?=w416:bool)
            n179 = case shown="True" w418 {
              frame False {
              }
              frame True {
                n180 = local write "Сегменты"(bool[] [TRUE, TRUE, TRUE, TRUE, TRUE, TRUE, TRUE, TRUE, TRUE, TRUE, TRUE, TRUE, TRUE, TRUE, TRUE, TRUE] ("Сегменты")) -> ()
              }
            }
            n181 = case shown="True" w416 {
              frame False {
              }
              frame True {
                n182 = local write "Сегменты"(bool[] [FALSE, FALSE, FALSE, FALSE, FALSE, FALSE, FALSE, FALSE, FALSE, FALSE, FALSE, FALSE, FALSE, FALSE, FALSE, FALSE] ("Сегменты")) -> ()
              }
            }
            n183 = stacked-sequence {
              tunnel: w415 -> [w421 _ _]
              frame #0 {
                n184 = local write "Command"(w421) -> ()
              }
              frame #1 {
                n185 = local write "Записать"(TRUE ("Записать")) -> ()
                n186 = Wait (ms)(milliseconds to wait=u32 1000) -> ()  [unwired: 1 out]
              }
              frame #2 {
                n187 = local write "Записать"(FALSE ("Записать")) -> ()
                n188 = Wait (ms)(milliseconds to wait=u32 1000) -> ()  [unwired: 1 out]
              }
            }
          }
        }
      }
    }
  }
  n189 = call <instrlib>:"niDMM Close.vi"("error in (no error)"=w29, "instrument handle"=w30) -> ()  [unwired: 9 in, 1 out]
  n190 = while {
    tunnel: [w432] -> w31
    tunnel: w34 -> [w430]
    tunnel: w33 -> [w429]
    tunnel: [w426] -> w32
    stop <- w428 stop-if-true
    # "Настройка вольтметра NI PXI-4071"
    n191 = Wait (ms)(milliseconds to wait=u32 1) -> ()  [unwired: 1 out]
    n192 = flat-sequence {
      tunnel: [w439] -> w434
      tunnel: w430 -> [w437]
      tunnel: w429 -> [w441]
      tunnel: [w438] -> w433
      tunnel: w434 -> [w450]
      tunnel: w433 -> [w453]
      tunnel: [w449] -> w428
      tunnel: [w448] -> w426
      tunnel: [w447] -> w427
      frame #0 {
        w435 = T5 6.5 items=["3 1/2"=3.5, "4 1/2"=4.5, "5 1/2"=5.5, "6 1/2"=6.5, "7 1/2"=7.5] ("Resolution in Digits")
        n193 = Fract/Exp String To Number(string="NI DMM 1 Voltage Range 4") -> (number=w440:dbl)  [unwired: 3 in, 1 out]
        n194 = call-poly <instrlib>:"niDMM Config Measurement.vi"("Range"=w440, "Resolution in Digits"=w435, "error in (no error)"=w441, "Function"=niDMM_Function."DC Volts" ("Measurement Type"), "instrument handle"=w437) -> ("error out"=w438:errorcluster, "instrument handle out"=w439:refnum<k15>)  [unwired: 5 in]
      }
      frame #1 {
        n195 = call <instrlib>:"niDMM Read.vi"("error in (no error)"=w453, "instrument handle"=w450) -> ("error out"=w447:errorcluster, "Measurement"=w445:dbl, "instrument handle out"=w448:refnum<k15>)  [unwired: 7 in]
        "Voltage, V" <- w445
        n196 = Fract/Exp String To Number(string="NI DMM 1 units 4") -> (number=w451:dbl)  [unwired: 3 in, 1 out]
        n197 = Multiply(x=w451, y=w445) -> (x*y=w443:dbl)
        n198 = Absolute Value(x=w443) -> (abs(x)=→"Voltage Char":dbl)
        n199 = Absolute Value(x=w443) -> (abs(x)=→"Voltage":dbl)
        n200 = local read "Стоп"() -> (w449:bool)
      }
    }
    n201 = call <vilib>:"Simple Error Handler.vi"("error in (no error)"=w427) -> ("error out"=w432:errorcluster)  [unwired: 1 in, 7 out]
  }
  n202 = invoke class="AmateurStepperMotor" method="Stop"(reference=w16) -> (reference out=w14:refnum<k24>, "Stop"=w15:refnum<k24>)  [unwired: 2 in, 1 out]
  n203 = property class="AmateurStepperMotor"(reference=w14, "HoldOn"=FALSE) -> (reference out=w13:refnum<k24>)  [unwired: 1 in, 1 out]
  n204 = invoke class="AmateurStepperMotor" method="Dispose"(reference=w13) -> (error out=w10:errorcluster)  [unwired: 2 in, 2 out]
  n205 = invoke class="SerialPort" method="Close"(reference=w9, error in=w10) -> (reference out=w8:refnum<k24>, error out=w11:errorcluster)  [unwired: 1 in, 1 out]
  n206 = invoke class="Task" method="Wait"(reference=w15) -> ()  [unwired: 2 in, 3 out]
  n207 = Close Reference(reference=w8, error in (no error)=w11) -> (error out=w12:errorcluster)
  n208 = call <vilib>:"Simple Error Handler.vi"("error in (no error)"=w12) -> ()  [unwired: 1 in, 8 out]
  n209 = call <instrlib>:"niDMM Close.vi"("error in (no error)"=w31, "instrument handle"=w32) -> ()  [unwired: 9 in, 1 out]
  n210 = call <instrlib>:"niDCPower Close.vi"("instrument handle"=w37) -> ()  [unwired: 10 in, 1 out]
  n211 = VISA Close(VISA resource name=w20, error in (no error)=w19) -> (error out=w21:errorcluster)
  n212 = call "Ophir Error Message.vi"("error in (no error)"=w21) -> ()  [unwired: 3 in, 4 out]
